vi "Write_MessageEmitter.vi"(8 "error in (no error)":errorcluster, 10 "Emitter":string, 11 "Messages in":refnum<class "Messages.lvclass">) -> (0 "error out":errorcluster, 3 "Messages out":refnum<class "Messages.lvclass">)   [LabVIEW 2013, in "Messages.lvclass"]
uses:
  Messages.lvclass
  Messages.lvclass/Messages.ctl
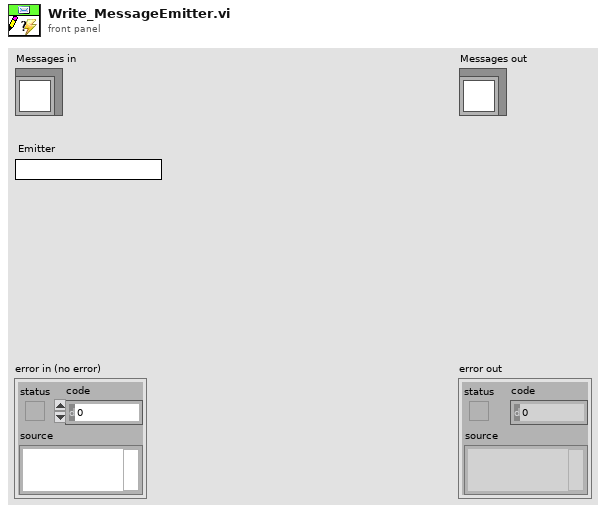
[diagram p1: front panel]
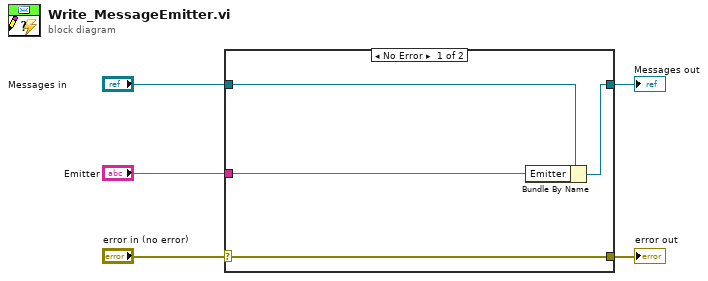
[diagram p0: block diagram]
diagram:
  n1 = case shown="No Error" "error in (no error)" {
    selector: "error in (no error)" -> [w9 w10]
    tunnel: [w9 w10] -> w4
    tunnel: [w7 w11] -> w2
    tunnel: "Messages in" -> [w8 w11]
    tunnel: "Emitter" -> [w6 _]
    frame No Error {
      n2 = Bundle By Name(cluster=w8, "Emitter"=w6) -> (w7:refnum<class "Messages.lvclass">)
    }
    frame Error {
    }
  }
  "error out" <- w4
  "Messages out" <- w2
